vi "get Analog Config Labview.vi"(6 "analogIndex":i32, 7 "pmuIndex":i32, 9 "pseudoPdcId":i32, 10 "name":string, 11 "analogCfg":T1) -> (1 "function return":i32, 2 "name out":string, 3 "analogCfg out":T1)   [LabVIEW 2013, in "C37118-DLL.lvlib" / "StrongridDLL.lvlib"]
doc: "STRONGRIDIEEEC37118DLL_API int __cdecl getAnalogConfigLabview(noArraysAnalogConfig *analogCfg, char* name, int32_t pseudoPdcId, int32_t pmuIndex, int32_t analogIndex);"
uses:
  StrongridDLL.lvlib
  StrongridDLL.dll
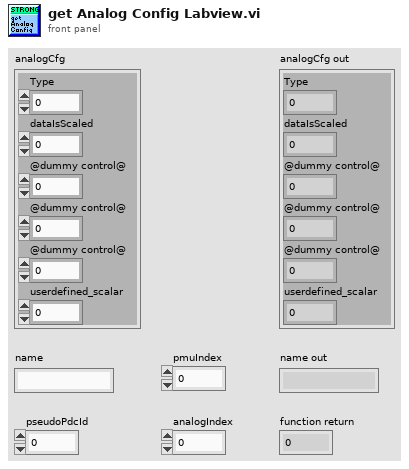
[diagram p1: front panel]
types:
  T1 = cluster{"Type":i32, "dataIsScaled":u8, "@dummy control@":i8, "@dummy control@":i8, "@dummy control@":i8, "userdefined_scalar":sgl}
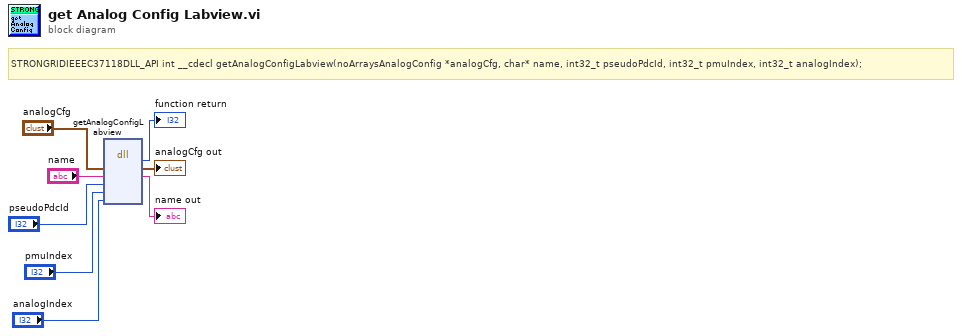
[diagram p0: block diagram]
diagram:
  # "STRONGRIDIEEEC37118DLL_API int __cdecl getAnalogConfigLabview(noArraysAnalogConfig *analogCfg, char* name, int32_t pseudoPdcId, int32_t pmuIndex, int32_t analogIndex);"
  n1 = dll-call lib="C:/dev/statnett/S3DK-Startup/LabVIEW PRL Library LV2013/c37118-dll/labview/vi/Auto Generated/StrongridDLL.*" fn="getAnalogConfigLabview"("analogCfg"="analogCfg", "name"="name", "pseudoPdcId"="pseudoPdcId", "pmuIndex"="pmuIndex", "analogIndex"="analogIndex") -> (→"function return":i32, "analogCfg"=→"analogCfg out":T1, "name"=→"name out":string)  [unwired: 6 in, 2 out]
